vi "RNN - Update Params.vi"(0 "learning_rate":dbl, 1 "dParams":T3, 3 "_params":T2) -> (8 "params_":T2)   [LabVIEW 2014]
uses:
  <vilib>/Analysis/Matrix/Datatypes/RealMatrix.ctl
  <vilib>/Analysis/Matrix/Numeric/Conversions/Matrix To Array - RM.vi
  <vilib>/Analysis/Matrix/Numeric/Conversions/Array To Matrix - RA2.vi
  <vilib>/Analysis/Matrix/Numeric/Add/Add - RM,RM.vi
  <vilib>/Analysis/Matrix/NI_Matrix.lvlib
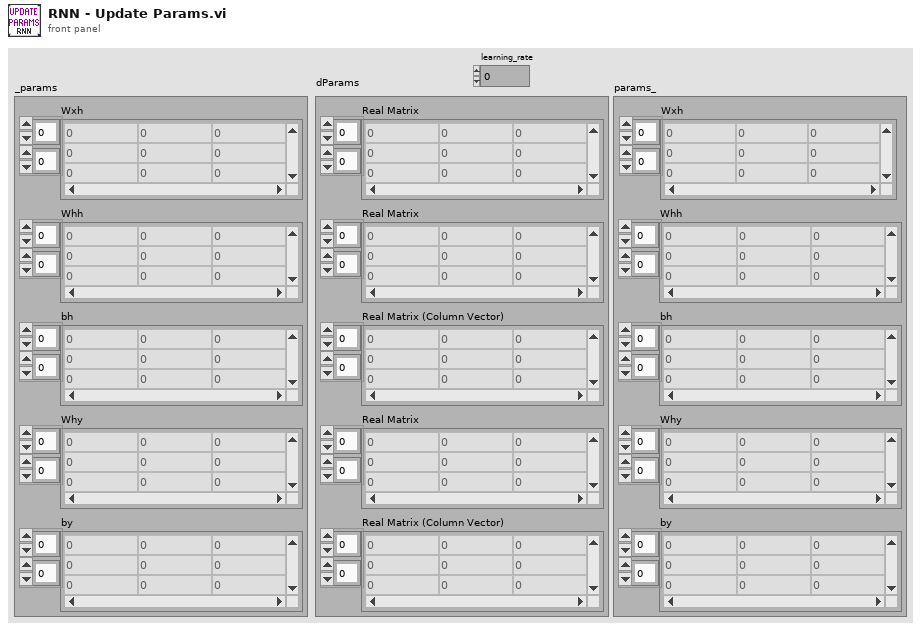
[diagram p1: front panel]
types:
  T1 = typedef "NI_Matrix.lvlib/RealMatrix.ctl" = dbl[][]
  T2 = cluster{"Wxh":T1, "Whh":T1, "bh":T1, "Why":T1, "by":T1}
  T3 = cluster{"Real Matrix":T1, "Real Matrix":T1, "Real Matrix (Column Vector)":T1, "Real Matrix":T1, "Real Matrix (Column Vector)":T1}
  T4 = cluster{"A + B":T1, "A + B":T1, "A + B":T1, "A + B":T1, "A + B":T1}
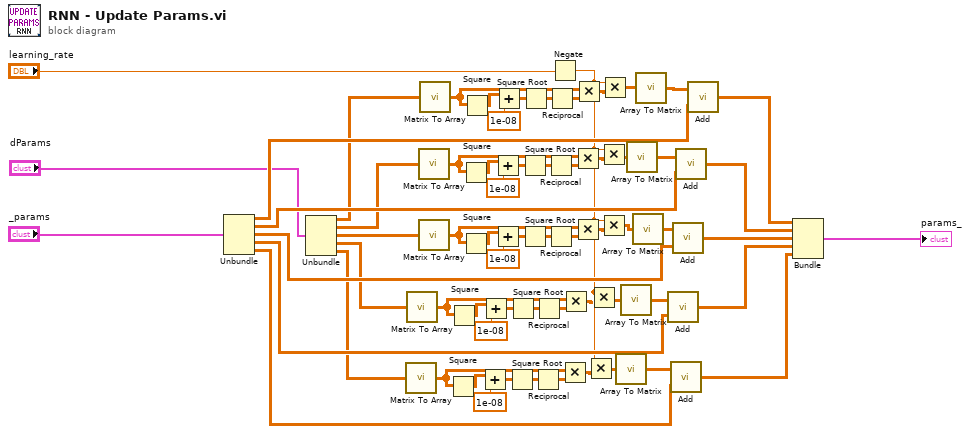
[diagram p0: block diagram]
diagram:
  n1 = Unbundle("_params") -> ("Wxh"=w51:T1, "Whh"=w52:T1, "bh"=w54:T1, "Why"=w56:T1, "by"=w58:T1)
  n2 = Unbundle("dParams") -> ("Real Matrix"=w45:T1, "Real Matrix"=w9:T1, "Real Matrix (Column Vector)"=w8:T1, "Real Matrix"=w7:T1, "Real Matrix (Column Vector)"=w6:T1)
  n3 = call-poly <vilib>:"Matrix To Array.vi"("Real Matrix"=w6) -> ("Real 2D Array"=w14:dbl[][])
  n4 = call-poly <vilib>:"Matrix To Array.vi"("Real Matrix"=w7) -> ("Real 2D Array"=w21:dbl[][])
  n5 = call-poly <vilib>:"Matrix To Array.vi"("Real Matrix"=w9) -> ("Real 2D Array"=w35:dbl[][])
  n6 = call-poly <vilib>:"Matrix To Array.vi"("Real Matrix"=w8) -> ("Real 2D Array"=w28:dbl[][])
  n7 = call-poly <vilib>:"Matrix To Array.vi"("Real Matrix"=w45) -> ("Real 2D Array"=w42:dbl[][])
  n8 = Square(x=w14) -> (x^2=w10:dbl[][])
  n9 = Square(x=w21) -> (x^2=w17:dbl[][])
  n10 = Square(x=w35) -> (x^2=w31:dbl[][])
  n11 = Square(x=w28) -> (x^2=w24:dbl[][])
  n12 = Square(x=w42) -> (x^2=w38:dbl[][])
  n13 = Add(x=w10, y=1e-08 ("x")) -> (x+y=w16:dbl[][])
  n14 = Add(x=w17, y=1e-08 ("x")) -> (x+y=w23:dbl[][])
  n15 = Add(x=w31, y=1e-08 ("x")) -> (x+y=w37:dbl[][])
  n16 = Add(x=w24, y=1e-08 ("x")) -> (x+y=w30:dbl[][])
  n17 = Add(x=w38, y=1e-08 ("x")) -> (x+y=w44:dbl[][])
  n18 = Square Root(x=w16) -> (sqrt(x)=w15:dbl[][])
  n19 = Square Root(x=w23) -> (sqrt(x)=w22:dbl[][])
  n20 = Square Root(x=w37) -> (sqrt(x)=w36:dbl[][])
  n21 = Square Root(x=w30) -> (sqrt(x)=w29:dbl[][])
  n22 = Square Root(x=w44) -> (sqrt(x)=w43:dbl[][])
  n23 = Reciprocal(x=w15) -> (1/x=w13:dbl[][])
  n24 = Reciprocal(x=w22) -> (1/x=w20:dbl[][])
  n25 = Reciprocal(x=w36) -> (1/x=w34:dbl[][])
  n26 = Reciprocal(x=w29) -> (1/x=w27:dbl[][])
  n27 = Reciprocal(x=w43) -> (1/x=w41:dbl[][])
  n28 = Negate(x="learning_rate") -> (-x=w48:dbl)
  n29 = Multiply(x=w14, y=w13) -> (x*y=w12:dbl[][])
  n30 = Multiply(x=w21, y=w20) -> (x*y=w19:dbl[][])
  n31 = Multiply(x=w35, y=w34) -> (x*y=w33:dbl[][])
  n32 = Multiply(x=w28, y=w27) -> (x*y=w26:dbl[][])
  n33 = Multiply(x=w42, y=w41) -> (x*y=w40:dbl[][])
  n34 = Multiply(x=w48, y=w12) -> (x*y=w4:dbl[][])
  n35 = Multiply(x=w48, y=w19) -> (x*y=w3:dbl[][])
  n36 = Multiply(x=w48, y=w33) -> (x*y=w1:dbl[][])
  n37 = Multiply(x=w48, y=w26) -> (x*y=w2:dbl[][])
  n38 = Multiply(x=w48, y=w40) -> (x*y=w5:dbl[][])
  n39 = call-poly <vilib>:"Array To Matrix.vi"("Real 2D Array"=w4) -> ("Real Matrix"=w59:T1)
  n40 = call-poly <vilib>:"Array To Matrix.vi"("Real 2D Array"=w3) -> ("Real Matrix"=w57:T1)
  n41 = call-poly <vilib>:"Array To Matrix.vi"("Real 2D Array"=w1) -> ("Real Matrix"=w53:T1)
  n42 = call-poly <vilib>:"Array To Matrix.vi"("Real 2D Array"=w2) -> ("Real Matrix"=w55:T1)
  n43 = call-poly <vilib>:"Array To Matrix.vi"("Real 2D Array"=w5) -> ("Real Matrix"=w50:T1)
  n44 = call-poly <vilib>:"Add.vi"("Real Matrix B"=w56, "Real Matrix A"=w57) -> ("A + B"=w63:T1)
  n45 = call-poly <vilib>:"Add.vi"("Real Matrix B"=w58, "Real Matrix A"=w59) -> ("A + B"=w64:T1)
  n46 = call-poly <vilib>:"Add.vi"("Real Matrix B"=w54, "Real Matrix A"=w55) -> ("A + B"=w62:T1)
  n47 = call-poly <vilib>:"Add.vi"("Real Matrix B"=w52, "Real Matrix A"=w53) -> ("A + B"=w61:T1)
  n48 = call-poly <vilib>:"Add.vi"("Real Matrix B"=w51, "Real Matrix A"=w50) -> ("A + B"=w60:T1)
  n49 = Bundle("A + B"=w60, "A + B"=w61, "A + B"=w62, "A + B"=w63, "A + B"=w64) -> (→"params_":T4)  [unwired: 1 in]
